vi "Write UploadSerialNumber.vi"(8 "error in (no error)":errorcluster, 10 "UploadSerialNumber":cluster{"Socket":i32, "SerialNumber":string}, 11 "Assert Event in":refnum<class "Assert Event.lvclass">) -> (0 "error out":errorcluster, 3 "Assert Event out":refnum<class "Assert Event.lvclass">)   [LabVIEW 2019, in "Assert.lvlib" / "Assert Event.lvclass"]
uses:
  Assert Event.lvclass
  Assert Event.lvclass/Assert Event.ctl
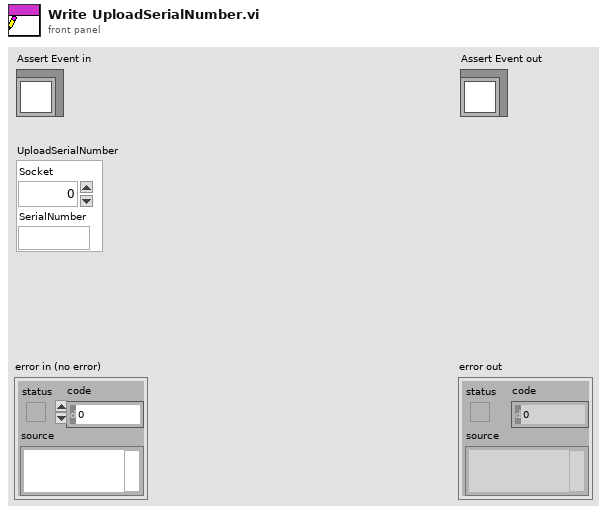
[diagram p1: front panel]
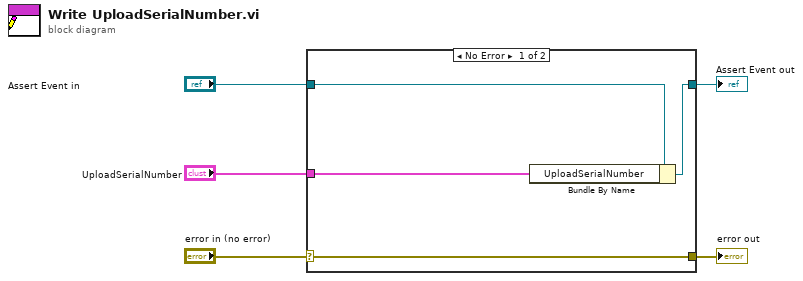
[diagram p0: block diagram]
diagram:
  n1 = case shown="No Error" "error in (no error)" {
    selector: "error in (no error)" -> [w9 w10]
    tunnel: [w9 w10] -> w4
    tunnel: [w7 w11] -> w2
    tunnel: "Assert Event in" -> [w8 w11]
    tunnel: "UploadSerialNumber" -> [w6 _]
    frame No Error {
      n2 = Bundle By Name(cluster=w8, "UploadSerialNumber"=w6) -> (w7:refnum<class "Assert Event.lvclass">)
    }
    frame Error {
    }
  }
  "error out" <- w4
  "Assert Event out" <- w2
